vi "Cycle 4 Main Spin.vi"(0 "GEA2 Reference In":refnum<k24>, 1 "Basket Speeds (rpm)":u32[](array[numeric])=[125, 450, 700], 5 "GEA Inputs":T1={"Source"=228, "Destination"=35} {"Destination" format="%.0x"; "Source" format="%.0x"}, 7 "Standalone?":bool, 9 "Dwell Times (s)":dbl[](array[numeric])=[90.0, 30.0, 600.0], 11 "Error In":errorcluster, 12 "Basket Speed Tolerance (rpm)":u32=2) -> (4 "GEA2 Reference Out":refnum<k24>, 6 "Pass/Fail?":bool, 8 "Report Text":string, 15 "Error Out":errorcluster)   [LabVIEW 2016, in "Centauro.lvlib"]
uses:
  Projects/Centauro.lvlib
  Q:/Common/DLLs/GEA3/GeaCommunication.dll
  Common/DLLs/GEA3/GeaCommunication.dll
  Common/LabVIEW GEA2 Toolkit/LabVIEW_GEA2_Toolkit.lvlibp/type defs/Source_Destination.ctl
  Common/LabVIEW GEA2 Toolkit/LabVIEW_GEA2_Toolkit.lvlibp/type defs/ERD Read Data In.ctl
  Common/LabVIEW GEA2 Toolkit/LabVIEW_GEA2_Toolkit.lvlibp/type defs/Data Type.ctl
  Valew Common/type defs/Drive Cycle Engine Request State.ctl
  Common/LabVIEW GEA2 Toolkit/LabVIEW_GEA2_Toolkit.lvlibp
panel:
  out "3":u16
  out "2":u16
  out "1":u16
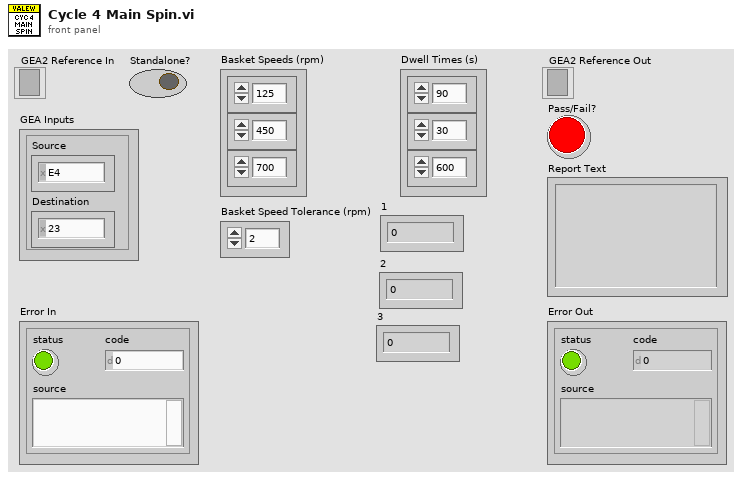
[diagram p1: front panel]
types:
  T1 = typedef "LabVIEW_GEA2_Toolkit.lvlibp/Source_Destination.ctl" = cluster{"Source":u8, "Destination":u8}
  T2 = typedef "Centauro.lvlib/Drive Cycle Engine Request State.ctl" = enum16{"Start", "Stop", "Pause", "Resume", "Select"}
  T3 = typedef "LabVIEW_GEA2_Toolkit.lvlibp/ERD Read Data In.ctl" = cluster{"ERD Number":u16, "Data Type":T4}
  T4 = typedef "LabVIEW_GEA2_Toolkit.lvlibp/Data Type.ctl" = enum16{"string", "boolean", "uint8_t", "uint16_t", "uint32_t", "uint64_t", "int8_t", "int16_t", "int32_t", "int64_t"}
  T5 = typedef "LabVIEW_GEA2_Toolkit.lvlibp/ERD Read Data Out.ctl" = cluster{"ERD Number":u16, "Data":string}
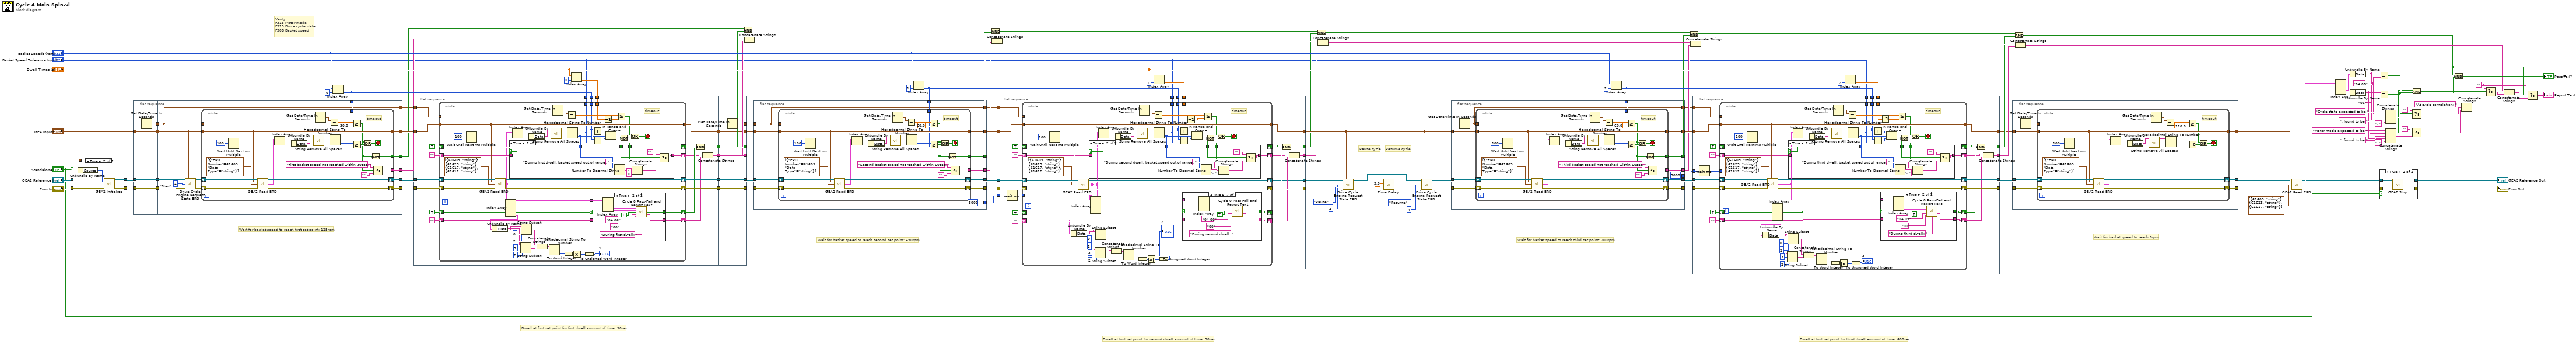
[diagram p0: block diagram]
diagram:
  w11 = ""
  w118 = "04 0B" ("y")
  w106 = "06" ("y")
  # "Wait for basket speed to reach 0rpm"
  # "Resume cycle"
  # "Pause cycle"
  # "Dwell at first set point for third dwell amount of time: 600sec"
  # "Wait for basket speed to reach third set point: 700rpm"
  # "Dwell at first set point for second dwell amount of time: 30sec"
  # "Wait for basket speed to reach second set point: 450rpm"
  # "Verify\nF313 Motor mode\nF319 Drive cycle state\nF30B Basket speed"
  # "Dwell at first set point for first dwell amount of time: 90sec"
  # "Wait for basket speed to reach first set point: 125rpm"
  n1 = case shown="True" "Standalone?" {
    tunnel: "GEA2 Reference In" -> [w125 _]
    tunnel: [w125 w130] -> w27
    tunnel: "Error In" -> [w124 w129]
    tunnel: [w124 w128] -> w28
    tunnel: "GEA Inputs" -> [_ w127]
    frame False {
    }
    frame True {
      n2 = Unbundle By Name(w127) -> ("Source"=w126:u8)
      n3 = call "GEA2 Initialize.vi"("Source Address"=w126, "error in"=w129) -> ("GEA2 Reference Out"=w130:refnum<k24>, "error out"=w128:errorcluster)  [unwired: 11 in, 1 out]
    }
  }
  n4 = flat-sequence {
    tunnel: "GEA Inputs" -> [w134]
    tunnel: [w134] -> w29
    tunnel: w28 -> [w131]
    tunnel: w27 -> [w132]
    tunnel: [w133] -> w26
    tunnel: [w132] -> w25
    tunnel: [w131] -> w24
    tunnel: [w148] -> w86
    tunnel: [w147] -> w87
    tunnel: [w146] -> w99
    tunnel: [w143] -> w52
    tunnel: [w144] -> w50
    tunnel: w68 -> [w145]
    tunnel: [w135] -> w32
    tunnel: w29 -> [w136]
    tunnel: w26 -> [w135]
    tunnel: w25 -> [w140]
    tunnel: w24 -> [w139]
    frame #0 {
      n5 = Get Date/Time In Seconds() -> (seconds since 1Jan1904=w133:timestamp)
    }
    frame #1 {
      n6 = call "Drive Cycle Engine Request State ERD.vi"("GEA2 Reference In"=w140, "GEA Inputs"=w136, "Cycle ID"=u8 4, "Drive Cycle Engine Request State"=Drive_Cycle_Engine_Request_State."Start", "Error In"=w139) -> ("GEA2 Reference Out"=w138:refnum<k24>, "Error Out"=w137:errorcluster)  [unwired: 9 in]
      n7 = while {
        shift-right: [w171] -> w148
        shift-left: w137 -> [w172]
        shift-right: [w169] -> w147
        shift-left: w138 -> [w170]
        tunnel: w136 -> [w167]
        tunnel: [w167] -> w146
        tunnel: w135 -> [w149]
        tunnel: w145 -> [w157]
        tunnel: [w152] -> w144
        tunnel: [w150] -> w143
        stop <- w164 stop-if-true
        # "timeout"
        n8 = Wait Until Next ms Multiple(millisecond multiple=u32 100 ("milliseconds to wait")) -> ()  [unwired: 1 out]
        n9 = call "GEA2 Read ERD.vi"("GEA2 Reference In"=w170, "GEA Inputs"=w167, "Read ERD List"=T3[] [{"ERD Number"=61609, "Data Type"=enum."string"}], "Error In"=w172) -> ("GEA2 Reference Out"=w169:refnum<k24>, "ERD Data Out"=w156:T5[], "Error Out"=w171:errorcluster)  [unwired: 8 in, 1 out]
        n10 = Index Array(array=w156) -> (element=w168:T5)  [unwired: 1 in]
        n11 = Unbundle By Name(w168) -> ("Data"=w160:string)
        n12 = call "String Remove All Spaces.vi"("Input String"=w160) -> ("Spaces Removed"=w161:string)  [unwired: 13 in, 1 out]
        n13 = Get Date/Time In Seconds() -> (seconds since 1Jan1904=w165:timestamp)
        n14 = Subtract(x=w165, y=w149) -> (x-y=w166:dbl)
        n15 = Hexadecimal String To Number(string=w161) -> (number=w159:u32)  [unwired: 2 in, 1 out]
        n16 = Greater Or Equal?(x=w166, y=30.0) -> (x >= y?=w151:bool)
        n17 = Greater Or Equal?(x=w159, y=w157) -> (x >= y?=w155:bool)
        n18 = Or(x=w151, y=w155) -> (x .or. y?=w164:bool)
        n19 = Not(x=w151) -> (.not. x?=w150:bool)
        n20 = Select(t="First basket speed not reached within 30sec. ", s=w151, f="") -> (s? t:f=w152:string)
      }
    }
  }
  n21 = Index Array(array="Basket Speeds (rpm)", index=0) -> (element=w68:u32)
  n22 = flat-sequence {
    tunnel: w89 -> [w185]
    tunnel: w68 -> [w184]
    tunnel: "Basket Speed Tolerance (rpm)" -> [w183]
    tunnel: w86 -> [w190]
    tunnel: w99 -> [w191]
    tunnel: w87 -> [w192]
    tunnel: w32 -> [w173]
    tunnel: [w188] -> w7
    tunnel: [w187] -> w6
    tunnel: [w186] -> w5
    tunnel: [w177] -> w4
    tunnel: [w174] -> w3
    tunnel: [w260] -> w8
    tunnel: [w261] -> w49
    tunnel: [w262] -> w51
    tunnel: [w263] -> w83
    tunnel: [w264] -> w85
    tunnel: [w265] -> w84
    tunnel: w7 -> [w265]
    tunnel: w6 -> [w264]
    tunnel: w5 -> [w263]
    tunnel: w4 -> [w262]
    tunnel: w3 -> [w261]
    frame #0 {
      n23 = while {
        shift-right: [w237] -> w188
        shift-left: w190 -> [w238]
        shift-right: [w235] -> w187
        shift-left: w192 -> [w236]
        tunnel: w191 -> [w233]
        tunnel: [w233] -> w186
        tunnel: w173 -> [w231]
        shift-right: [w215] -> w178
        shift-left: TRUE -> [w217]
        tunnel: w185 -> [w208]
        tunnel: w184 -> [w222]
        tunnel: w183 -> [w221]
        shift-right: [w219] -> w175
        shift-left: "" -> [w216]
        shift-right: [w209] -> w179
        shift-left: TRUE -> [w212]
        shift-right: [w210] -> w176
        shift-left: "" -> [w211]
        stop <- w229 stop-if-true
        # "timeout"
        n24 = Wait Until Next ms Multiple(millisecond multiple=u32 100 ("milliseconds to wait")) -> ()  [unwired: 1 out]
        n25 = call "GEA2 Read ERD.vi"("GEA2 Reference In"=w236, "GEA Inputs"=w233, "Read ERD List"=T3[] [{"ERD Number"=61609, "Data Type"=enum."string"}, {"ERD Number"=61623, "Data Type"=enum."string"}, {"ERD Number"=61617, "Data Type"=enum."string"}, {"ERD Number"=61612, "Data Type"=enum."string"}], "Error In"=w238) -> ("GEA2 Reference Out"=w235:refnum<k24>, "ERD Data Out"=w206:T5[], "Error Out"=w237:errorcluster)  [unwired: 8 in, 1 out]
        n26 = Index Array(array=w206) -> (element #4=w205:T5)  [unwired: 4 in, 3 out]
        n27 = Unbundle By Name(w205) -> ("Data"=w193:string)
        n28 = Index Array(array=w206) -> (element=w234:T5)  [unwired: 1 in]
        n29 = String Subset(string=w193, offset (0)=3, length (rest)=2 ("length (rest)")) -> (substring=w201:string)
        n30 = String Subset(string=w193, offset (0)=0, length (rest)=2 ("length (rest)")) -> (substring=w200:string)
        n31 = Unbundle By Name(w234) -> ("Data"=w225:string)
        n32 = Concatenate Strings(w200, w201) -> (w195:string)
        n33 = Hexadecimal String To Number(string=w195) -> (number=w204:u32)  [unwired: 2 in, 1 out]
        n34 = call "String Remove All Spaces.vi"("Input String"=w225) -> ("Spaces Removed"=w226:string)  [unwired: 13 in, 1 out]
        n35 = Get Date/Time In Seconds() -> (seconds since 1Jan1904=w230:timestamp)
        n36 = To Word Integer(number=w204) -> (16bit integer=w203:i16)
        n37 = Subtract(x=w230, y=w231) -> (x-y=w232:dbl)
        n38 = Hexadecimal String To Number(string=w226) -> (number=w220:u32)  [unwired: 2 in, 1 out]
        n39 = Absolute Value(x=w203) -> (abs(x)=w202:i16)
        n40 = To Unsigned Word Integer(number=w202) -> (unsigned 16bit integer=→"1":u16)
        n41 = case shown="True" w212 {
          selector: w212 -> [w239 _]
          tunnel: w211 -> [w240 _]
          tunnel: [w240 w248] -> w210
          tunnel: [w239 w249] -> w209
          tunnel: w206 -> [_ w247]
          frame False {
          }
          frame True {
            n42 = Index Array(array=w247) -> (element #2=w245:T5, element #3=w244:T5)  [unwired: 3 in, 1 out]
            n43 = call "Cycle 0 Pass-Fail and Report Text.vi"("Drive Cycle State"=w245, "Motor Mode"=w244, "Previous Pass/Fail"=TRUE, "Cycle State Expected"="04 06", "Motor Mode Expected"="00", "Header"="During first dwell: ") -> ("Pass/Fail?"=w249:bool, "Report Text"=w248:string)  [unwired: 8 in]
          }
        }
        n44 = Add(x=w222, y=w221) -> (x+y=w224:u32)
        n45 = Subtract(x=w222, y=w221) -> (x-y=w223:u32)
        n46 = Decrement(x=w208) -> (x-1=w207:dbl)
        n47 = In Range and Coerce(upper limit=w224, x=w220, lower limit=w223) -> (In Range?=w218:bool)  [unwired: 1 out]
        n48 = case shown="True" w217 {
          selector: w217 -> [w250 _]
          tunnel: w220 -> [_ w257]
          tunnel: [w251 w254] -> w219
          tunnel: w218 -> [_ w253]
          tunnel: w216 -> [w251 _]
          tunnel: [w250 w253] -> w215
          frame False {
          }
          frame True {
            n49 = Number To Decimal String(number=w257) -> (decimal integer string=w256:string)  [unwired: 1 in]
            n50 = Concatenate Strings("During first dwell, basket speed out of range: " ("string"), w256, ". " ("string")) -> (w255:string)
            n51 = Select(t="", s=w253, f=w255) -> (s? t:f=w254:string)
          }
        }
        n52 = Greater Or Equal?(x=w232, y=w207) -> (x >= y?=w213:bool)
        n53 = Not(x=w218) -> (.not. x?=w214:bool)
        n54 = Or(x=w213, y=w214) -> (x .or. y?=w229:bool)
      }
      n55 = And(x=w178, y=w179) -> (x .and. y?=w177:bool)
      n56 = Concatenate Strings(w175, w176) -> (w174:string)
    }
    frame #1 {
      n57 = Get Date/Time In Seconds() -> (seconds since 1Jan1904=w260:timestamp)
    }
  }
  n58 = Index Array(array="Dwell Times (s)", index=0) -> (element=w89:dbl)
  n59 = And(x=w52, y=w51) -> (x .and. y?=w48:bool)
  n60 = Concatenate Strings(w50, w49) -> (w47:string)
  n61 = flat-sequence {
    tunnel: [w273] -> w81
    tunnel: [w272] -> w80
    tunnel: [w271] -> w79
    tunnel: [w268] -> w45
    tunnel: [w269] -> w46
    tunnel: w78 -> [w270]
    tunnel: w84 -> [w274]
    tunnel: w83 -> [w275]
    tunnel: w85 -> [w276]
    tunnel: [w267] -> w31
    tunnel: w8 -> [w267]
    tunnel: [u32 3000 ("milliseconds to wait")] -> w1
    frame #0 {
      n62 = while {
        shift-right: [w299] -> w273
        shift-left: w274 -> [w300]
        shift-right: [w297] -> w272
        shift-left: w276 -> [w298]
        tunnel: w275 -> [w295]
        tunnel: [w295] -> w271
        tunnel: w267 -> [w277]
        tunnel: w270 -> [w285]
        tunnel: [w280] -> w269
        tunnel: [w278] -> w268
        stop <- w292 stop-if-true
        # "timeout"
        n63 = Wait Until Next ms Multiple(millisecond multiple=u32 100 ("milliseconds to wait")) -> ()  [unwired: 1 out]
        n64 = call "GEA2 Read ERD.vi"("GEA2 Reference In"=w298, "GEA Inputs"=w295, "Read ERD List"=T3[] [{"ERD Number"=61609, "Data Type"=enum."string"}], "Error In"=w300) -> ("GEA2 Reference Out"=w297:refnum<k24>, "ERD Data Out"=w284:T5[], "Error Out"=w299:errorcluster)  [unwired: 8 in, 1 out]
        n65 = Index Array(array=w284) -> (element=w296:T5)  [unwired: 1 in]
        n66 = Unbundle By Name(w296) -> ("Data"=w288:string)
        n67 = call "String Remove All Spaces.vi"("Input String"=w288) -> ("Spaces Removed"=w289:string)  [unwired: 13 in, 1 out]
        n68 = Get Date/Time In Seconds() -> (seconds since 1Jan1904=w293:timestamp)
        n69 = Subtract(x=w293, y=w277) -> (x-y=w294:dbl)
        n70 = Hexadecimal String To Number(string=w289) -> (number=w287:u32)  [unwired: 2 in, 1 out]
        n71 = Greater Or Equal?(x=w294, y=60.0) -> (x >= y?=w279:bool)
        n72 = Greater Or Equal?(x=w287, y=w285) -> (x >= y?=w283:bool)
        n73 = Or(x=w279, y=w283) -> (x .or. y?=w292:bool)
        n74 = Not(x=w279) -> (.not. x?=w278:bool)
        n75 = Select(t="Second basket speed not reached within 60sec. ", s=w279, f="") -> (s? t:f=w280:string)
      }
    }
  }
  n76 = Index Array(array="Basket Speeds (rpm)", index=1) -> (element=w78:u32)
  n77 = And(x=w48, y=w45) -> (x .and. y?=w42:bool)
  n78 = Concatenate Strings(w47, w46) -> (w43:string)
  n79 = flat-sequence {
    tunnel: [w318] -> w62
    tunnel: [w317] -> w53
    tunnel: [w308] -> w41
    tunnel: [w305] -> w44
    tunnel: w76 -> [w316]
    tunnel: w78 -> [w315]
    tunnel: "Basket Speed Tolerance (rpm)" -> [w314]
    tunnel: w81 -> [w320]
    tunnel: w79 -> [w321]
    tunnel: w80 -> [w322]
    tunnel: [w304] -> w63
    tunnel: w31 -> [w303]
    tunnel: w1 -> [w302]
    frame #0 {
      n80 = Wait (ms)(milliseconds to wait=w302) -> (millisecond timer value=w301:u32)
      n81 = while {
        shift-right: [w367] -> w318
        shift-left: w320 -> [w368]
        shift-right: [w365] -> w304
        shift-left: w322 -> [w366]
        tunnel: w321 -> [w363]
        tunnel: [w363] -> w317
        tunnel: w303 -> [w361]
        shift-right: [w346] -> w309
        shift-left: TRUE -> [w348]
        tunnel: w316 -> [w339]
        tunnel: w315 -> [w353]
        tunnel: w314 -> [w352]
        shift-right: [w350] -> w306
        shift-left: "" -> [w347]
        shift-right: [w340] -> w310
        shift-left: TRUE -> [w343]
        shift-right: [w341] -> w307
        shift-left: "" -> [w342]
        tunnel: w301 -> [_]
        stop <- w359 stop-if-true
        # "timeout"
        n82 = Wait Until Next ms Multiple(millisecond multiple=u32 100) -> ()  [unwired: 1 out]
        n83 = call "GEA2 Read ERD.vi"("GEA2 Reference In"=w366, "GEA Inputs"=w363, "Read ERD List"=T3[] [{"ERD Number"=61609, "Data Type"=enum."string"}, {"ERD Number"=61623, "Data Type"=enum."string"}, {"ERD Number"=61617, "Data Type"=enum."string"}, {"ERD Number"=61612, "Data Type"=enum."string"}], "Error In"=w368) -> ("GEA2 Reference Out"=w365:refnum<k24>, "ERD Data Out"=w337:T5[], "Error Out"=w367:errorcluster)  [unwired: 8 in, 1 out]
        n84 = Index Array(array=w337) -> (element #4=w336:T5)  [unwired: 4 in, 3 out]
        n85 = Unbundle By Name(w336) -> ("Data"=w325:string)
        n86 = String Subset(string=w325, offset (0)=3, length (rest)=2 ("length (rest)")) -> (substring=w332:string)
        n87 = String Subset(string=w325, offset (0)=0, length (rest)=2 ("length (rest)")) -> (substring=w331:string)
        n88 = Index Array(array=w337) -> (element=w364:T5)  [unwired: 1 in]
        n89 = Concatenate Strings(w331, w332) -> (w326:string)
        n90 = Unbundle By Name(w364) -> ("Data"=w356:string)
        n91 = Hexadecimal String To Number(string=w326) -> (number=w335:u32)  [unwired: 2 in, 1 out]
        n92 = call "String Remove All Spaces.vi"("Input String"=w356) -> ("Spaces Removed"=w357:string)  [unwired: 13 in, 1 out]
        n93 = To Word Integer(number=w335) -> (16bit integer=w334:i16)
        n94 = Get Date/Time In Seconds() -> (seconds since 1Jan1904=w360:timestamp)
        n95 = Absolute Value(x=w334) -> (abs(x)=w333:i16)
        n96 = Subtract(x=w360, y=w361) -> (x-y=w362:dbl)
        n97 = Hexadecimal String To Number(string=w357) -> (number=w351:u32)  [unwired: 2 in, 1 out]
        n98 = To Unsigned Word Integer(number=w333) -> (unsigned 16bit integer=→"2":u16)
        n99 = Add(x=w353, y=w352) -> (x+y=w355:u32)
        n100 = Subtract(x=w353, y=w352) -> (x-y=w354:u32)
        n101 = case shown="True" w343 {
          selector: w343 -> [w369 _]
          tunnel: w342 -> [w370 _]
          tunnel: [w370 w378] -> w341
          tunnel: [w369 w379] -> w340
          tunnel: w337 -> [_ w377]
          frame False {
          }
          frame True {
            n102 = Index Array(array=w377) -> (element #2=w375:T5, element #3=w374:T5)  [unwired: 3 in, 1 out]
            n103 = call "Cycle 0 Pass-Fail and Report Text.vi"("Drive Cycle State"=w375, "Motor Mode"=w374, "Previous Pass/Fail"=TRUE, "Cycle State Expected"="04 06", "Motor Mode Expected"="00", "Header"="During second dwell: ") -> ("Pass/Fail?"=w379:bool, "Report Text"=w378:string)  [unwired: 8 in]
          }
        }
        n104 = Decrement(x=w339) -> (x-1=w338:dbl)
        n105 = In Range and Coerce(upper limit=w355, x=w351, lower limit=w354) -> (In Range?=w349:bool)  [unwired: 1 out]
        n106 = case shown="True" w348 {
          selector: w348 -> [w380 _]
          tunnel: w351 -> [_ w387]
          tunnel: [w381 w384] -> w350
          tunnel: w349 -> [_ w383]
          tunnel: w347 -> [w381 _]
          tunnel: [w380 w383] -> w346
          frame False {
          }
          frame True {
            n107 = Number To Decimal String(number=w387) -> (decimal integer string=w386:string)  [unwired: 1 in]
            n108 = Concatenate Strings("During second dwell, basket speed out of range: " ("string"), w386, ". " ("string")) -> (w385:string)
            n109 = Select(t="", s=w383, f=w385) -> (s? t:f=w384:string)
          }
        }
        n110 = Greater Or Equal?(x=w362, y=w338) -> (x >= y?=w344:bool)
        n111 = Not(x=w349) -> (.not. x?=w345:bool)
        n112 = Or(x=w344, y=w345) -> (x .or. y?=w359:bool)
      }
      n113 = And(x=w309, y=w310) -> (x .and. y?=w308:bool)
      n114 = Concatenate Strings(w306, w307) -> (w305:string)
    }
  }
  n115 = Index Array(array="Dwell Times (s)", index=1) -> (element=w76:dbl)
  n116 = And(x=w42, y=w41) -> (x .and. y?=w40:bool)
  n117 = Concatenate Strings(w43, w44) -> (w39:string)
  n118 = call "Drive Cycle Engine Request State ERD.vi"("GEA2 Reference In"=w63, "GEA Inputs"=w53, "Cycle ID"=u8 4, "Drive Cycle Engine Request State"=Drive_Cycle_Engine_Request_State."Pause", "Error In"=w62) -> ("GEA2 Reference Out"=w56:refnum<k24>, "Error Out"=w61:errorcluster)  [unwired: 9 in]
  n119 = call "Time Delay"("error in (no error)"=w61, "Delay Time (s)"=3.0) -> ("error out"=w57:errorcluster)  [unwired: 9 in]
  n120 = call "Drive Cycle Engine Request State ERD.vi"("GEA2 Reference In"=w56, "GEA Inputs"=w53, "Cycle ID"=u8 4, "Drive Cycle Engine Request State"=Drive_Cycle_Engine_Request_State."Resume", "Error In"=w57) -> ("GEA2 Reference Out"=w54:refnum<k24>, "Error Out"=w58:errorcluster)  [unwired: 9 in]
  n121 = flat-sequence {
    tunnel: [w397] -> w74
    tunnel: [w396] -> w73
    tunnel: [w395] -> w72
    tunnel: [w392] -> w37
    tunnel: [w393] -> w38
    tunnel: w71 -> [w394]
    tunnel: w58 -> [w398]
    tunnel: w53 -> [w399]
    tunnel: w54 -> [w400]
    tunnel: [w391] -> w30
    tunnel: [u32 3000 ("milliseconds to wait")] -> w2
    frame #0 {
      n122 = Get Date/Time In Seconds() -> (seconds since 1Jan1904=w391:timestamp)
      n123 = while {
        shift-right: [w423] -> w397
        shift-left: w398 -> [w424]
        shift-right: [w421] -> w396
        shift-left: w400 -> [w422]
        tunnel: w399 -> [w419]
        tunnel: [w419] -> w395
        tunnel: w391 -> [w401]
        tunnel: w394 -> [w409]
        tunnel: [w404] -> w393
        tunnel: [w402] -> w392
        stop <- w416 stop-if-true
        # "timeout"
        n124 = Wait Until Next ms Multiple(millisecond multiple=u32 100 ("milliseconds to wait")) -> ()  [unwired: 1 out]
        n125 = call "GEA2 Read ERD.vi"("GEA2 Reference In"=w422, "GEA Inputs"=w419, "Read ERD List"=T3[] [{"ERD Number"=61609, "Data Type"=enum."string"}], "Error In"=w424) -> ("GEA2 Reference Out"=w421:refnum<k24>, "ERD Data Out"=w408:T5[], "Error Out"=w423:errorcluster)  [unwired: 8 in, 1 out]
        n126 = Index Array(array=w408) -> (element=w420:T5)  [unwired: 1 in]
        n127 = Unbundle By Name(w420) -> ("Data"=w412:string)
        n128 = call "String Remove All Spaces.vi"("Input String"=w412) -> ("Spaces Removed"=w413:string)  [unwired: 13 in, 1 out]
        n129 = Get Date/Time In Seconds() -> (seconds since 1Jan1904=w417:timestamp)
        n130 = Subtract(x=w417, y=w401) -> (x-y=w418:dbl)
        n131 = Hexadecimal String To Number(string=w413) -> (number=w411:u32)  [unwired: 2 in, 1 out]
        n132 = Greater Or Equal?(x=w418, y=60.0) -> (x >= y?=w403:bool)
        n133 = Greater Or Equal?(x=w411, y=w409) -> (x >= y?=w407:bool)
        n134 = Or(x=w403, y=w407) -> (x .or. y?=w416:bool)
        n135 = Not(x=w403) -> (.not. x?=w402:bool)
        n136 = Select(t="Third basket speed not reached within 60sec. ", s=w403, f="") -> (s? t:f=w404:string)
      }
    }
  }
  n137 = Index Array(array="Basket Speeds (rpm)", index=2) -> (element=w71:u32)
  n138 = And(x=w40, y=w37) -> (x .and. y?=w36:bool)
  n139 = Concatenate Strings(w39, w38) -> (w35:string)
  n140 = flat-sequence {
    tunnel: [w442] -> w22
    tunnel: [w441] -> w23
    tunnel: [w440] -> w21
    tunnel: [w431] -> w33
    tunnel: [w428] -> w34
    tunnel: w69 -> [w439]
    tunnel: w71 -> [w438]
    tunnel: "Basket Speed Tolerance (rpm)" -> [w437]
    tunnel: w74 -> [w444]
    tunnel: w72 -> [w445]
    tunnel: w73 -> [w446]
    tunnel: w30 -> [w427]
    tunnel: w2 -> [w426]
    frame #0 {
      n141 = Wait (ms)(milliseconds to wait=w426) -> (millisecond timer value=w425:u32)
      n142 = while {
        shift-right: [w491] -> w442
        shift-left: w444 -> [w492]
        shift-right: [w489] -> w441
        shift-left: w446 -> [w490]
        tunnel: w445 -> [w487]
        tunnel: [w487] -> w440
        tunnel: w427 -> [w485]
        shift-right: [w469] -> w432
        shift-left: TRUE -> [w471]
        tunnel: w439 -> [w462]
        tunnel: w438 -> [w476]
        tunnel: w437 -> [w475]
        shift-right: [w473] -> w429
        shift-left: "" -> [w470]
        shift-right: [w463] -> w433
        shift-left: TRUE -> [w466]
        shift-right: [w464] -> w430
        shift-left: "" -> [w465]
        tunnel: w425 -> [_]
        stop <- w483 stop-if-true
        # "timeout"
        n143 = Wait Until Next ms Multiple(millisecond multiple=u32 100 ("milliseconds to wait")) -> ()  [unwired: 1 out]
        n144 = call "GEA2 Read ERD.vi"("GEA2 Reference In"=w490, "GEA Inputs"=w487, "Read ERD List"=T3[] [{"ERD Number"=61609, "Data Type"=enum."string"}, {"ERD Number"=61623, "Data Type"=enum."string"}, {"ERD Number"=61617, "Data Type"=enum."string"}, {"ERD Number"=61612, "Data Type"=enum."string"}], "Error In"=w492) -> ("GEA2 Reference Out"=w489:refnum<k24>, "ERD Data Out"=w460:T5[], "Error Out"=w491:errorcluster)  [unwired: 8 in, 1 out]
        n145 = Index Array(array=w460) -> (element #4=w455:T5)  [unwired: 4 in, 3 out]
        n146 = Unbundle By Name(w455) -> ("Data"=w448:string)
        n147 = String Subset(string=w448, offset (0)=3, length (rest)=2 ("length (rest)")) -> (substring=w454:string)
        n148 = String Subset(string=w448, offset (0)=0, length (rest)=2 ("length (rest)")) -> (substring=w453:string)
        n149 = Index Array(array=w460) -> (element=w488:T5)  [unwired: 1 in]
        n150 = Concatenate Strings(w453, w454) -> (w447:string)
        n151 = Unbundle By Name(w488) -> ("Data"=w479:string)
        n152 = Hexadecimal String To Number(string=w447) -> (number=w458:u32)  [unwired: 2 in, 1 out]
        n153 = To Word Integer(number=w458) -> (16bit integer=w457:i16)
        n154 = call "String Remove All Spaces.vi"("Input String"=w479) -> ("Spaces Removed"=w480:string)  [unwired: 13 in, 1 out]
        n155 = Get Date/Time In Seconds() -> (seconds since 1Jan1904=w484:timestamp)
        n156 = Absolute Value(x=w457) -> (abs(x)=w456:i16)
        n157 = Subtract(x=w484, y=w485) -> (x-y=w486:dbl)
        n158 = Hexadecimal String To Number(string=w480) -> (number=w474:u32)  [unwired: 2 in, 1 out]
        n159 = To Unsigned Word Integer(number=w456) -> (unsigned 16bit integer=→"3":u16)
        n160 = Add(x=w476, y=w475) -> (x+y=w478:u32)
        n161 = Subtract(x=w476, y=w475) -> (x-y=w477:u32)
        n162 = Decrement(x=w462) -> (x-1=w461:dbl)
        n163 = case shown="True" w466 {
          selector: w466 -> [w493 _]
          tunnel: w465 -> [w494 _]
          tunnel: [w494 w502] -> w464
          tunnel: [w493 w503] -> w463
          tunnel: w460 -> [_ w501]
          frame False {
          }
          frame True {
            n164 = Index Array(array=w501) -> (element #2=w499:T5, element #3=w498:T5)  [unwired: 3 in, 1 out]
            n165 = call "Cycle 0 Pass-Fail and Report Text.vi"("Drive Cycle State"=w499, "Motor Mode"=w498, "Previous Pass/Fail"=TRUE, "Cycle State Expected"="04 09", "Motor Mode Expected"="00", "Header"="During third dwell: ") -> ("Pass/Fail?"=w503:bool, "Report Text"=w502:string)  [unwired: 8 in]
          }
        }
        n166 = In Range and Coerce(upper limit=w478, x=w474, lower limit=w477) -> (In Range?=w472:bool)  [unwired: 1 out]
        n167 = case shown="True" w471 {
          selector: w471 -> [w504 _]
          tunnel: w474 -> [_ w511]
          tunnel: [w505 w508] -> w473
          tunnel: w472 -> [_ w507]
          tunnel: w470 -> [w505 _]
          tunnel: [w504 w507] -> w469
          frame False {
          }
          frame True {
            n168 = Number To Decimal String(number=w511) -> (decimal integer string=w510:string)  [unwired: 1 in]
            n169 = Concatenate Strings("During third dwell, basket speed out of range: " ("string"), w510, ". " ("string")) -> (w509:string)
            n170 = Select(t="", s=w507, f=w509) -> (s? t:f=w508:string)
          }
        }
        n171 = Greater Or Equal?(x=w486, y=w461) -> (x >= y?=w467:bool)
        n172 = Not(x=w472) -> (.not. x?=w468:bool)
        n173 = Or(x=w467, y=w468) -> (x .or. y?=w483:bool)
      }
      n174 = And(x=w432, y=w433) -> (x .and. y?=w431:bool)
      n175 = Concatenate Strings(w429, w430) -> (w428:string)
    }
  }
  n176 = Index Array(array="Dwell Times (s)", index=2) -> (element=w69:dbl)
  n177 = flat-sequence {
    tunnel: [w516] -> w18
    tunnel: [w515] -> w19
    tunnel: [w514] -> w20
    tunnel: w22 -> [w518]
    tunnel: w21 -> [w519]
    tunnel: w23 -> [w520]
    frame #0 {
      n178 = Get Date/Time In Seconds() -> (seconds since 1Jan1904=w517:timestamp)
      n179 = while {
        shift-right: [w538] -> w516
        shift-left: w518 -> [w539]
        shift-right: [w536] -> w515
        shift-left: w520 -> [w537]
        tunnel: w519 -> [w534]
        tunnel: [w534] -> w514
        tunnel: w517 -> [w521]
        stop <- w531 stop-if-true
        # "timeout"
        n180 = Wait Until Next ms Multiple(millisecond multiple=u32 100 ("milliseconds to wait")) -> ()  [unwired: 1 out]
        n181 = call "GEA2 Read ERD.vi"("GEA2 Reference In"=w537, "GEA Inputs"=w534, "Read ERD List"=T3[] [{"ERD Number"=61609, "Data Type"=enum."string"}], "Error In"=w539) -> ("GEA2 Reference Out"=w536:refnum<k24>, "ERD Data Out"=w524:T5[], "Error Out"=w538:errorcluster)  [unwired: 8 in, 1 out]
        n182 = Index Array(array=w524) -> (element=w535:T5)  [unwired: 1 in]
        n183 = Unbundle By Name(w535) -> ("Data"=w527:string)
        n184 = call "String Remove All Spaces.vi"("Input String"=w527) -> ("Spaces Removed"=w528:string)  [unwired: 13 in, 1 out]
        n185 = Get Date/Time In Seconds() -> (seconds since 1Jan1904=w532:timestamp)
        n186 = Subtract(x=w532, y=w521) -> (x-y=w533:dbl)
        n187 = Hexadecimal String To Number(string=w528) -> (number=w526:u32)  [unwired: 2 in, 1 out]
        n188 = Greater Or Equal?(x=w533, y=120.0) -> (x >= y?=w522:bool)
        n189 = Equal To 0?(x=w526) -> (x = 0?=w523:bool)
        n190 = Or(x=w522, y=w523) -> (x .or. y?=w531:bool)
      }
    }
  }
  n191 = And(x=w36, y=w33) -> (x .and. y?=w12:bool)
  n192 = Concatenate Strings(w35, w34) -> (w14:string)
  n193 = call "GEA2 Read ERD.vi"("GEA2 Reference In"=w19, "GEA Inputs"=w20, "Read ERD List"=T3[] [{"ERD Number"=61609, "Data Type"=enum."string"}, {"ERD Number"=61623, "Data Type"=enum."string"}, {"ERD Number"=61617, "Data Type"=enum."string"}], "Error In"=w18) -> ("GEA2 Reference Out"=w93:refnum<k24>, "ERD Data Out"=w120:T5[], "Error Out"=w95:errorcluster)  [unwired: 8 in, 1 out]
  n194 = Index Array(array=w120) -> (element #2=w123:T5, element #3=w122:T5)  [unwired: 3 in, 1 out]
  n195 = Unbundle By Name(w123) -> ("Data"=w116:string)
  n196 = Unbundle By Name(w122) -> ("Data"=w104:string)
  n197 = Equal?(x=w116, y=w118) -> (x = y?=w113:bool)
  n198 = Equal?(x=w104, y=w106) -> (x = y?=w112:bool)
  n199 = case shown="True" "Standalone?" {
    tunnel: [w540 w544] -> w96
    tunnel: w95 -> [w540 w543]
    tunnel: w93 -> [w541 w542]
    tunnel: [w541 _] -> w92
    frame False {
    }
    frame True {
      n200 = call "GEA2 Stop.vi"("GEA2 Reference In"=w542, "Error In"=w543) -> ("Error Out"=w544:errorcluster)  [unwired: 13 in]
    }
  }
  "GEA2 Reference Out" <- w92
  "Error Out" <- w96
  n201 = Concatenate Strings("Cycle state expected to be " ("string"), w118, ", found to be " ("string"), w116, ". " ("string")) -> (w114:string)
  n202 = Concatenate Strings("Motor mode expected to be " ("string"), w106, ", found to be " ("string"), w104, ". " ("string")) -> (w109:string)
  n203 = And(x=w112, y=w113) -> (x .and. y?=w16:bool)
  n204 = Select(t="", s=w113, f=w114) -> (s? t:f=w102:string)
  n205 = Select(t="", s=w112, f=w109) -> (s? t:f=w101:string)
  n206 = And(x=w12, y=w16) -> (x .and. y?=→"Pass/Fail?":bool)
  n207 = Concatenate Strings("At cycle completion: " ("string"), w102, w101) -> (w108:string)
  n208 = Select(t=w11, s=w16, f=w108) -> (s? t:f=w13:string)
  n209 = Concatenate Strings(w14, w13) -> (w10:string)
  n210 = Select(t=w11, s=w12, f=w10) -> (s? t:f=→"Report Text":string)
